vi "INIdouble.vi"(7 "Section":string, 8 "error in (no error)":errorcluster, 9 "default value":dbl, 10 "Key":string, 11 "Refnum in":T1) -> (0 "Error Out":errorcluster, 3 "Refnum out":T1)   [LabVIEW 2013]
uses:
  <vilib>/Utility/config.llb/Config Data RefNum.ctl
  <vilib>/Utility/config.llb/Read Key (Double).vi
  <vilib>/Utility/config.llb/Write Key (Double).vi
  <vilib>/Utility/config.llb/NI_LVConfig.lvlib
panel:
  out "Value":dbl
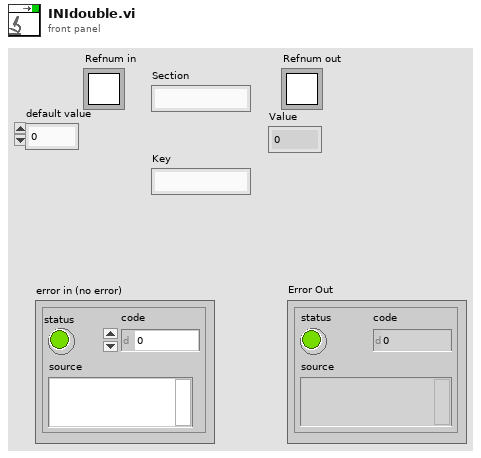
[diagram p1: front panel]
types:
  T1 = typedef "NI_LVConfig.lvlib/Config Data RefNum.ctl" = refnum<k1>
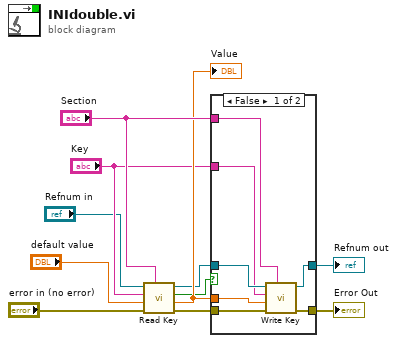
[diagram p0: block diagram]
diagram:
  n1 = call-poly <vilib>:"Read Key.vi"("section"="Section", "error in (no error)"="error in (no error)", "default value"="default value", "key"="Key", "refnum"="Refnum in") -> ("error out"=w5:errorcluster, "value"=w9:dbl, "found?"=w3:bool, "refnum out"=w4:T1)  [unwired: 3 in]
  "Value" <- w9
  n2 = case shown="False" w3 {
    tunnel: [w17 w20] -> w10
    tunnel: w4 -> [w18 w20]
    tunnel: w9 -> [w16 _]
    tunnel: w5 -> [w15 w19]
    tunnel: [w14 w19] -> w2
    tunnel: "Section" -> [w13 _]
    tunnel: "Key" -> [w12 _]
    frame False {
      n3 = call-poly <vilib>:"Write Key.vi"("section"=w13, "error in (no error)"=w15, "value"=w16, "key"=w12, "refnum"=w18) -> ("error out"=w14:errorcluster, "refnum out"=w17:T1)  [unwired: 4 in, 1 out]
    }
    frame True {
    }
  }
  "Refnum out" <- w10
  "Error Out" <- w2
